vi "extract_initialize_hw.vi"(5 "multipart message in":string[](array[string]), 11 "error in (no error)":errorcluster) -> (6 "Mode":T2, 8 "hwclass":T1, 10 "Valid Message?":bool, 14 "Debug info":string, 15 "error out":errorcluster)   [LabVIEW 2019, in "mmW_commands.lvlib"]
doc: "- Extract_message (command specific)\no Validate parameters , JSON format and also command-specific parameters' formats and values\no Extract parameters from JSON to cluster (or directly to indicators\no Validate data field\no Extract data (if there is any…e.g at write_tx command)"
uses:
  mmW_commands.lvlib
  typedefs/mode.ctl
  typedefs/instr_hwclass.ctl
  Instrument Parameters.ctl
  typedefs/ports.ctl
  typedefs/burst_mode.ctl
  <vilib>/addons/_JKI.lib/Serialization/JSON/JKI JSON Serialization.lvlib
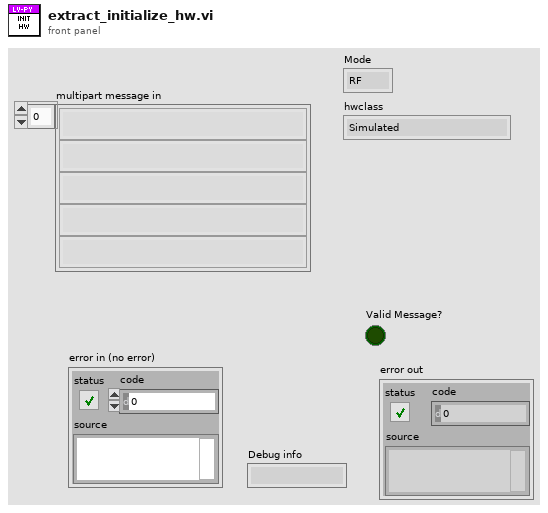
[diagram p1: front panel]
types:
  T1 = typedef "mmW_commands.lvlib/instr_hwclass.ctl" = enum16{"Simulated", "NI_mmW01", "Other"}
  T2 = typedef "mmW_commands.lvlib/mode.ctl" = enum16{"RF", "IF", "BB"}
  T3 = typedef "mmW_commands.lvlib/Instrument Parameters.ctl" = cluster{"Write TX":cluster{"burstname":string, "burst_length":dbl}, "configure_fs":cluster{"port":T4, "fs":dbl}, "configure_rf":cluster{"port":T4, "fc":dbl, "gain":dbl}, "initialize_hw":cluster{"mode":T2, "hwclass":T1}, "start":cluster{"acq_length":dbl, "bursts":string[]}, "trigger_burst":cluster{"burst_mode":T5, "bursts":string[]}, "trigger_sync_enable":cluster{"Enable":bool}, "lo_sync_enable":cluster{"Enable":bool}, "equalization_enable":cluster{"Enable":bool}, "transceive":cluster{"burstname":string, "burst_mode":T5, "bursts":string[], "acq_length":dbl}, "generic_no_param":cluster{"no_param":string}}
  T4 = typedef "mmW_commands.lvlib/ports.ctl" = enum16{"rx", "tx"}
  T5 = typedef "mmW_commands.lvlib/burst_mode.ctl" = enum16{"burst", "continuous"}
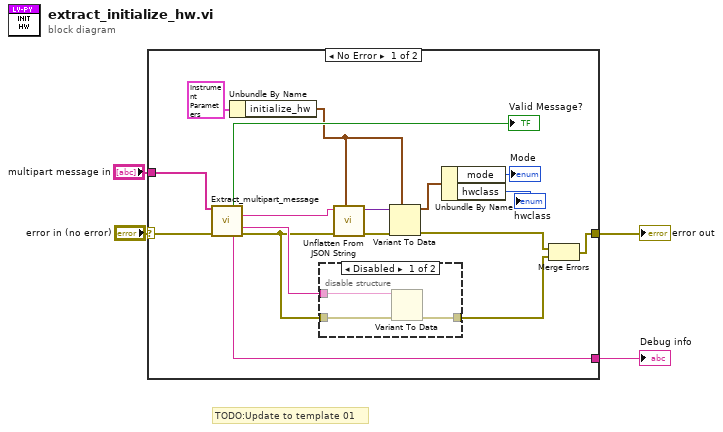
[diagram p0: block diagram]
diagram:
  # "TODO:Update to template 01"
  n1 = case shown="No Error" "error in (no error)" {
    selector: "error in (no error)" -> [w21 w26]
    tunnel: [w9 w26] -> w4
    tunnel: "multipart message in" -> [w5 _]
    tunnel: [w19 _] -> w1
    frame No Error {
      n2 = call "Extract_multipart_message.vi"("multipart message in"=w5, "error in (no error)"=w21) -> ("Valid message?"=→"Valid Message?":bool, "parameters"=w18:string, "data out"=w13:string, "Debug info"=w19:string, "error out"=w12:errorcluster)  [unwired: 6 in, 3 out]
      n3 = Unbundle By Name(T3 {"Write TX"={"burstname"="", "burst_length"=0.0}, "configure_fs"={"port"=enum."rx", "fs"=0.0}, "configure_rf"={"port"=enum."rx", "fc"=0.0, "gain"=0.0}, "initialize_hw"={"mode"=enum."RF", "hwclass"=enum."Simulated"}, "start"={"acq_length"=1000.0, "bursts"=[]}, "trigger_burst"={"burst_mode"=enum."burst", "bursts"=[]}, "trigger_sync_enable"={"Enable"=FALSE}, "lo_sync_enable"={"Enable"=FALSE}, "equalization_enable"={"Enable"=FALSE}, "transceive"={"burstname"="", "burst_mode"=enum."burst", "bursts"=[], "acq_length"=1000.0}, "generic_no_param"={"no_param"=""}} ("Instrument parameters")) -> ("initialize_hw"=w7:cluster{"mode":T2, "hwclass":T1})
      n4 = disable-structure shown="Disabled" {
        disable-tunnel: w13 -> [w24 _]
        disable-tunnel: w12 -> [w23 w25]
        disable-tunnel: [w22 w25] -> w10
        frame Disabled {
          n5 = Variant To Data(error in=w23, Variant=w24) -> (error out=w22:errorcluster)  [unwired: 1 in, 1 out]
        }
        frame Enabled {
        }
      }
      n6 = call <vilib>:"Unflatten From JSON String.vi"("Type and Defaults"=w7, "error in (no error)"=w12, "JSON String"=w18) -> ("error out"=w17:errorcluster, "Variant"=w16:variant)  [unwired: 7 in]
      n7 = Variant To Data(error in=w17, type=w7, Variant=w16) -> (data=w15:cluster{"mode":T2, "hwclass":T1}, error out=w11:errorcluster)
      n8 = Unbundle By Name(w15) -> ("mode"=→"Mode":T2, "hwclass"=→"hwclass":T1)
      n9 = Merge Errors(w11, w10) -> (w9:errorcluster)
    }
    frame Error {
    }
  }
  "error out" <- w4
  "Debug info" <- w1
